vi "curve fit.vi"(8 "Curve fit":enum16{"Exponential", "Logarithm"}(ring), 9 "day":i32, 10 "X":i32[](array[numeric]), 11 "Y":i32[](array[numeric])) -> (1 "damping":dbl, 2 "amplitude":dbl, 3 "Cluster":cluster{i32[], dbl[]}, 4 "offset":dbl)   [LabVIEW 2019]
uses:
  <vilib>/Analysis/NI_AALPro.lvlib
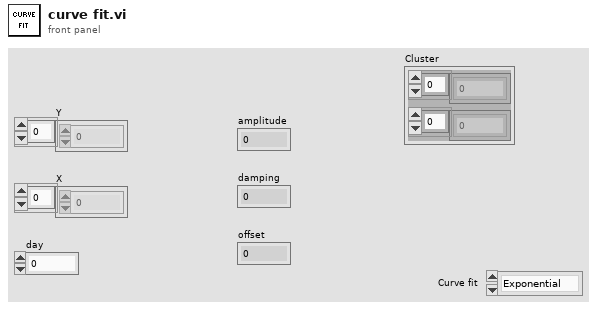
[diagram p1: front panel]
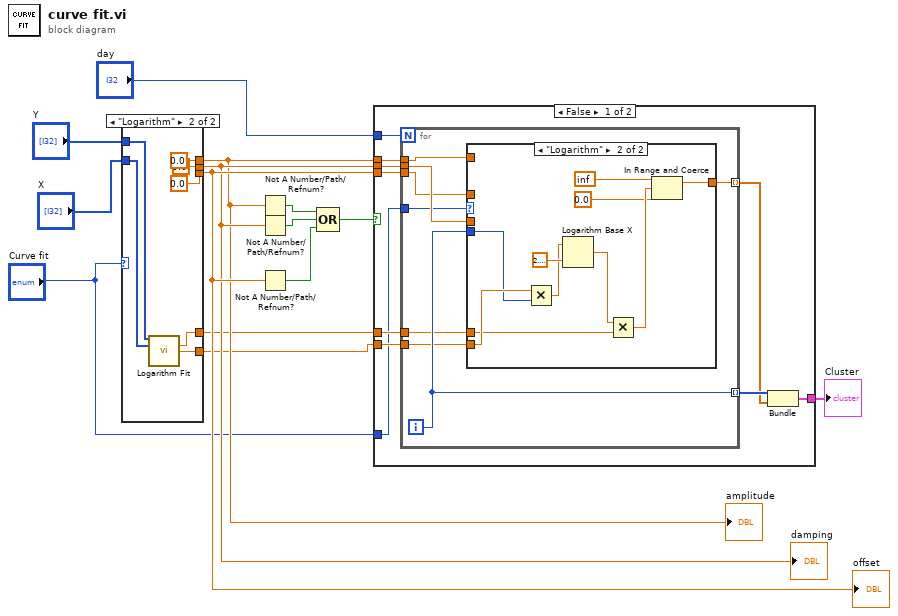
[diagram p0: block diagram]
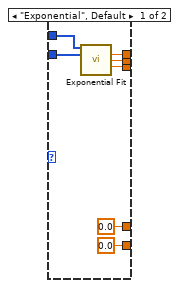
[diagram p2: hidden frame]
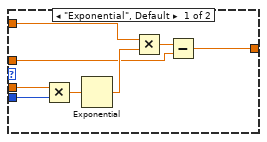
[diagram p3: hidden frame]
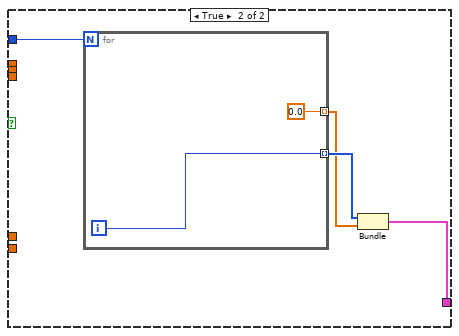
[diagram p4: hidden frame]
diagram:
  n1 = case shown="\"Logarithm\"" "Curve fit" {
    tunnel: [w21 0.0 ("offset")] -> w13
    tunnel: [w20 0.0 ("damping")] -> w12
    tunnel: [w19 0.0 ("amplitude")] -> w11
    tunnel: "X" -> [w18 w22]
    tunnel: "Y" -> [w17 w23]
    tunnel: [0.0 ("amplitude") w28] -> w3
    tunnel: [0.0 ("scale") w27] -> w2
    frame "Exponential", Default {
      n2 = call <vilib>:"Exponential Fit.vi"("Y"=w17, "X"=w18) -> ("amplitude"=w19:dbl, "damping"=w20:dbl, "offset"=w21:dbl)  [unwired: 8 in, 3 out]
    }
    frame "Logarithm" {
      n3 = call <vilib>:"Logarithm Fit.vi"("Y"=w23, "X"=w22) -> ("amplitude"=w28:dbl, "scale"=w27:dbl)  [unwired: 9 in, 3 out]
    }
  }
  "offset" <- w13
  "damping" <- w12
  "amplitude" <- w11
  n4 = Not A Number/Path/Refnum?(number/path/refnum=w11) -> (NaN/Path/Refnum?=w5:bool)
  n5 = Not A Number/Path/Refnum?(number/path/refnum=w12) -> (NaN/Path/Refnum?=w6:bool)
  n6 = Not A Number/Path/Refnum?(number/path/refnum=w13) -> (NaN/Path/Refnum?=w7:bool)
  n7 = Compound Arithmetic op=OR(w5, w6, w7) -> (w8:bool)
  n8 = case shown="False" w8 {
    tunnel: w11 -> [w37 _]
    tunnel: w12 -> [w36 _]
    tunnel: w13 -> [w35 _]
    tunnel: "day" -> [w34 w68]
    tunnel: [w32 w65] -> w4
    tunnel: w3 -> [w31 _]
    tunnel: w2 -> [w30 _]
    tunnel: "Curve fit" -> [w29 _]
    frame False {
      n9 = for {
        N: w34 -> [_]
        tunnel: w37 -> [w45]
        tunnel: w36 -> [w46]
        tunnel: w35 -> [w44]
        tunnel: [w43] -> w33 mode=indexing
        tunnel: [w42] -> w38 mode=indexing
        tunnel: w31 -> [w41]
        tunnel: w30 -> [w40]
        tunnel: w29 -> [w39]
        i -> [w42]
        n10 = case shown="\"Logarithm\"" w39 {
          tunnel: w46 -> [w54 _]
          tunnel: w45 -> [w51 _]
          tunnel: w44 -> [w49 _]
          tunnel: [w48 w55] -> w43
          tunnel: w42 -> [w47 w62]
          tunnel: w41 -> [_ w59]
          tunnel: w40 -> [_ w63]
          frame "Exponential", Default {
            n11 = Multiply(x=w54, y=w47) -> (x*y=w53:dbl)
            n12 = Exponential(1:w53) -> (0:w52:dbl)
            n13 = Multiply(x=w51, y=w52) -> (x*y=w50:dbl)
            n14 = Subtract(x=w50, y=w49) -> (x-y=w48:dbl)
          }
          frame "Logarithm" {
            n15 = Multiply(x=w63, y=w62) -> (x*y=w61:dbl)
            n16 = Logarithm Base X(1:2.718281828459045, 2:w61) -> (0:w60:dbl)
            n17 = Multiply(x=w60, y=w59) -> (x*y=w57:dbl)
            n18 = In Range and Coerce(upper limit=inf, x=w57, lower limit=0.0) -> (coerced(x)=w55:dbl)  [unwired: 1 out]
          }
        }
      }
      n19 = Bundle(w38, w33) -> (w32:cluster{i32[], dbl[]})  [unwired: 1 in]
    }
    frame True {
      n20 = for {
        N: w68 -> [_]
        tunnel: [w69] -> w67 mode=indexing
        tunnel: [0.0] -> w66 mode=indexing
        i -> [w69]
      }
      n21 = Bundle(w67, w66) -> (w65:cluster{i32[], dbl[]})  [unwired: 1 in]
    }
  }
  "Cluster" <- w4
